vi "CloseServer.vi"(3 "ROS":T1={"topic port"=0, "Node"="", "topic"="", "type"="", "node port"=0, "error "={"status"=FALSE, "code"=0, "source"=""}, "Direction"=enum."Node", "APIs"=[], "Update (ms)"=1, "write queue"=1}) -> (0 "error out":errorcluster)   [LabVIEW 2012]
doc: "Sends a message to the queue to unregister the server with the master."
uses:
  SubVIs/_ROSDirection.ctl
  SubVIs/_ROSControl.ctl
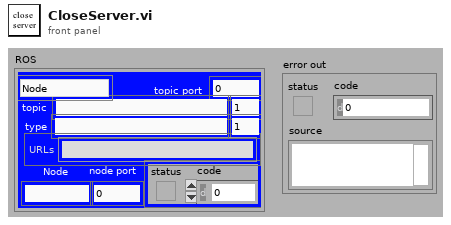
[diagram p1: front panel]
types:
  T1 = typedef "_ROSControl.ctl" = cluster{"topic port":u16, "Node":string, "topic":string, "type":string, "node port":u32, "error ":errorcluster, "Direction":T2, "APIs":string[], "Update (ms)":u16, "write queue":u16}
  T2 = typedef "_ROSDirection.ctl" = enum16{"Node", "Publisher", "Subscriber", "Service Client"}
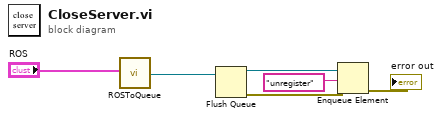
[diagram p0: block diagram]
diagram:
  n1 = call "ROSToQueue.vi"("ROS"="ROS") -> ("queue"=w4:refnum<queue>)  [unwired: 3 in, 1 out]
  n2 = Flush Queue(queue=w4) -> (queue out=w6:refnum<queue>, error out=w1:errorcluster)  [unwired: 1 in, 1 out]
  n3 = Enqueue Element(queue=w6, element="unregister", error in (no error)=w1) -> (error out=→"error out":errorcluster)  [unwired: 1 in, 2 out]
